vi "U32 to [U8].vi"(11 "Numeric":u32) -> (3 "output array":u8[](array[numeric]))   [LabVIEW 2016, in "IgusMotorDrive.lvclass"]
uses:
  IgusMotorDrive.lvclass
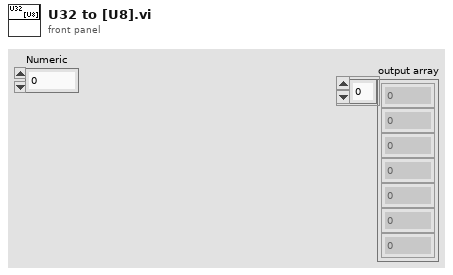
[diagram p1: front panel]
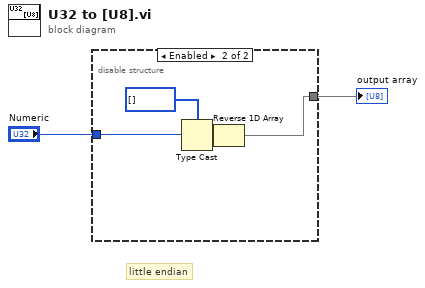
[diagram p0: block diagram]
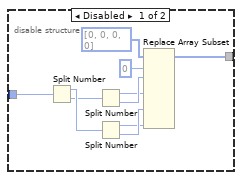
[diagram p2: hidden frame]
diagram:
  # "little endian"
  n1 = disable-structure shown="Enabled" {
    disable-tunnel: "Numeric" -> [w10 w14]
    disable-tunnel: [w3 w13] -> w1
    frame Disabled {
      n2 = Split Number(x=w10) -> (hi(x)=w9:u16, lo(x)=w8:u16)
      n3 = Split Number(x=w8) -> (hi(x)=w6:u8, lo(x)=w7:u8)
      n4 = Split Number(x=w9) -> (hi(x)=w4:u8, lo(x)=w5:u8)
      n5 = Replace Array Subset(array=u8[] [0, 0, 0, 0] ("Data [1-4]"), new element #1=w7, index #1=0 ("index"), new element #2=w6, new element #3=w5, new element #4=w4) -> (w3:u8[])  [unwired: 3 in]
    }
    frame Enabled {
      n6 = Type Cast(type=u8[] [] ("output array"), x=w14) -> (*(type *) &x=w15:u8[])
      n7 = Reverse 1D Array(array=w15) -> (reversed array=w13:u8[])
    }
  }
  "output array" <- w1
